vi "Event Trigger.vi"(11 "Boolean":bool=TRUE) -> (2 "State Passthrough":bool, 3 "Event Trigger":bool)   [LabVIEW 2016]
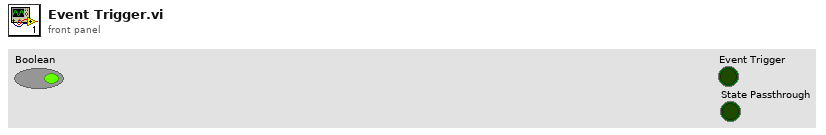
[diagram p1: front panel]
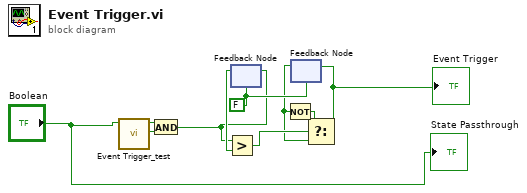
[diagram p0: block diagram]
diagram:
  w8 = FALSE ("Boolean")
  n1 = call "Event Trigger_test.vi"("Boolean"="Boolean") -> ("State Passthrough"=w2:bool, "Event Trigger"=w3:bool)  [unwired: 9 in]
  n2 = And(x=w3, y=w2) -> (x .and. y?=w1:bool)
  n3 = feedback-in #1(w1) -> ()
  n4 = feedback #1(w8) -> (w10:bool)
  n5 = Greater?(x=w1, y=w10) -> (0:w9:bool)
  n6 = feedback #2(w8) -> (w7:bool)
  n7 = Not(x=w7) -> (.not. x?=w6:bool)
  n8 = Select(t=w6, s=w9, f=w7) -> (s? t:f=w5:bool)
  "Event Trigger" <- w5
  n9 = feedback-in #2(w5) -> ()
  "State Passthrough" <- "Boolean"
